vi "AuMT8852B Carrier Drift Extended Results Query.vi"(7 "Stage":T1(ring), 8 "error in (no error)":errorcluster, 11 "VISA session":refnum<visa-resource-name>) -> (0 "error out":errorcluster, 2 "error code":i32, 3 "VISA session out":refnum<visa-resource-name>, 4 "Results":T2 {"DH5 results"."Average drift (kHz)" format="%.2f"; "DH5 results"."Max drift (kHz)" format="%.2f"; "DH5 results"."Max rate" format="%.2f"; "DH3 results"."Average drift (kHz)" format="%.2f"; "DH3 results"."Max drift (kHz)" format="%.2f"; "DH3 results"."Max rate" format="%.2f"; "DH1 results"."Average drift (kHz)" format="%.2f"; "DH1 results"."Max drift (kHz)" format="%.2f"; "DH1 results"."Max rate" format="%.2f"})   [LabVIEW 2017]
doc: "Anritsu MT8852B Bluetooth Tester\n\nReturns the results of the Carrier Drift test.\n\nINPUTS\nStage - results of the individual hopping stages of the test.\n\nOUTPUTS\nResults - measurements made during the test."
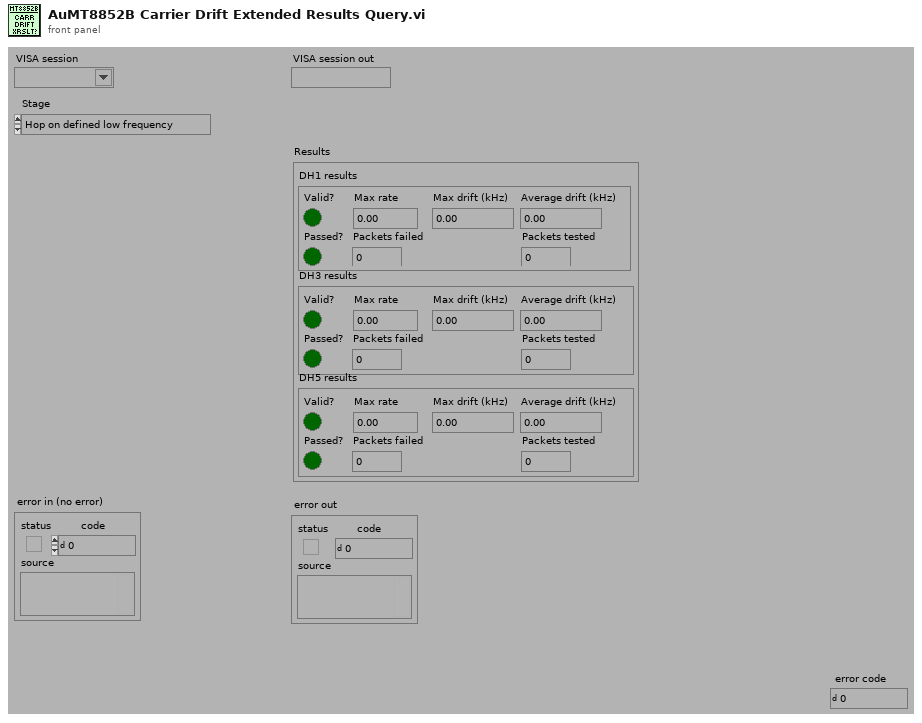
[diagram p1: front panel]
types:
  T1 = enum16{"Hop on defined low frequency", "Hop on defined medium frequency", "Hop on defined high frequency", "Hop on all channels", "Hop on any channels", "Hop off low frequency", "Hop off medium frequency", "Hop off high frequency"}
  T2 = cluster{"DH1 results":cluster{"Valid?":bool, "Max rate":dbl, "Max drift (kHz)":dbl, "Average drift (kHz)":dbl, "Packets failed":i32, "Packets tested":i32, "Passed?":bool}, "DH3 results":cluster{"Valid?":bool, "Max rate":dbl, "Max drift (kHz)":dbl, "Average drift (kHz)":dbl, "Packets failed":i32, "Packets tested":i32, "Passed?":bool}, "DH5 results":cluster{"Valid?":bool, "Max rate":dbl, "Max drift (kHz)":dbl, "Average drift (kHz)":dbl, "Packets failed":i32, "Packets tested":i32, "Passed?":bool}}
  T3 = enum16{"Simulate", "Range check", "Cache", "Query instrument status"}
  T4 = cluster{"[0]":cluster{bool, dbl, dbl, dbl, i32, i32, bool}, "[1]":cluster{bool, dbl, dbl, dbl, i32, i32, bool}, "[2]":cluster{bool, dbl, dbl, dbl, i32, i32, bool}}
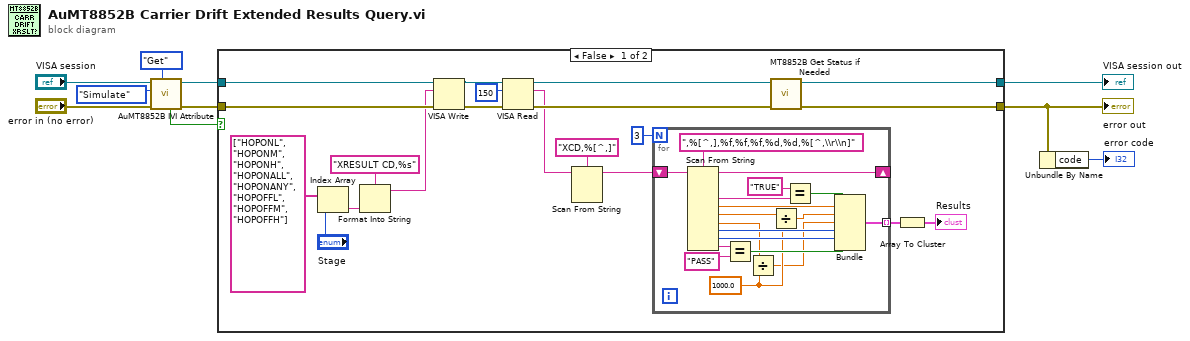
[diagram p0: block diagram]
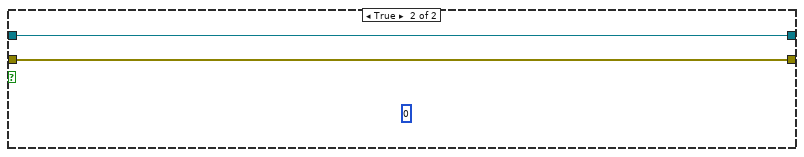
[diagram p2: hidden frame]
diagram:
  n1 = call <instrlib>:"AuMT8852B IVI Attribute.vi"("Set/Get (Set)"=enum16{"Set", "Get"}."Get", "error in (no error)"="error in (no error)", "Flag (Simulate)"=T3."Simulate", "VISA session"="VISA session") -> ("error out"=w7:errorcluster, "VISA session out"=w9:refnum<visa-resource-name>, "Value out"=w3:bool)  [unwired: 5 in]
  n2 = case shown="False" w3 {
    tunnel: [w25 w50] -> w10
    tunnel: [w24 w49] -> w1
    tunnel: w9 -> [w30 w50]
    tunnel: w7 -> [w29 w49]
    frame False {
      n3 = Index Array(array=string[] ["HOPONL", "HOPONM", "HOPONH", "HOPONALL", "HOPONANY", "HOPOFFL", "HOPOFFM", "HOPOFFH"], index="Stage") -> (element=w19:string)
      n4 = Format Into String(format string="XRESULT CD,%s" ("write buffer (\"\")"), w19) -> (resulting string=w17:string)  [unwired: 2 in, 1 out]
      n5 = VISA Write(VISA resource name=w30, write buffer=w17, error in (no error)=w29) -> (VISA resource name out=w28:refnum<visa-resource-name>, error out=w27:errorcluster)  [unwired: 1 out]
      n6 = VISA Read(VISA resource name=w28, byte count=u32 150 ("byte count (0)"), error in (no error)=w27) -> (VISA resource name out=w23:refnum<visa-resource-name>, read buffer=w12:string, error out=w22:errorcluster)  [unwired: 1 out]
      n7 = Scan From String(format string="XCD,%[^,]", input string=w12) -> (remaining string=w13:string)  [unwired: 4 in, 2 out]
      n8 = for {
        N: 3 -> [_]
        tunnel: [w38] -> w14 mode=indexing
        shift-right: [w36] -> _
        shift-left: w13 -> [w37]
        w32 = 1000.0 ("y")
        n9 = Scan From String(format string=",%[^,],%f,%f,%f,%d,%d,%[^,\\r\\n]", input string=w37) -> (remaining string=w36:string, output 1=w47:string, output 2=w42:dbl, output 3=w35:dbl, output 4=w33:dbl, output 5=w41:i32, output 6=w40:i32, output 7=w44:string)  [unwired: 9 in, 2 out]
        n10 = Equal?(x=w44, y="PASS") -> (x = y?=w39:bool)
        n11 = Divide(x=w33, y=w32) -> (x/y=w31:dbl)
        n12 = Divide(x=w35, y=w32) -> (x/y=w34:dbl)
        n13 = Equal?(x="TRUE", y=w47) -> (x = y?=w43:bool)
        n14 = Bundle(w43, w42, w34, w31, w41, w40, w39) -> (w38:cluster{bool, dbl, dbl, dbl, i32, i32, bool})  [unwired: 1 in]
      }
      n15 = call <instrlib>:"MT8852B Get Status if Needed.vi"("error in (no error)"=w22, "VISA session"=w23) -> ("error out"=w24:errorcluster, "VISA session out"=w25:refnum<visa-resource-name>)  [unwired: 8 in]
      n16 = Array To Cluster(array=w14) -> (cluster=→"Results":T4)
    }
    frame True {
      (unwired) u8 0
    }
  }
  "error out" <- w1
  "VISA session out" <- w10
  n17 = Unbundle By Name(w1) -> ("code"=→"error code":i32)
